vi "Facade.vi"(0 "Data In":T6, 2 "Display State In":T4, 3 "Container State":T5) -> (6 "Data Out":T6, 7 "Display State Out":T4, 8 "Action":T3)   [LabVIEW 2016, in "Queued Listbox.xctl"]
uses:
  Queued Listbox.xctl
  Data.ctl
  <vilib>/_xctls/Container State.ctl
  State.ctl
  <vilib>/_xctls/Action.ctl
  Menu object array.ctl
  Menu object.ctl
  <vilib>/_xctls/XControlSupport.lvlib
panel:
  out "Error Out":errorcluster
  in  "Menu object array":T1 {"Object name" items=["Select one..."]}
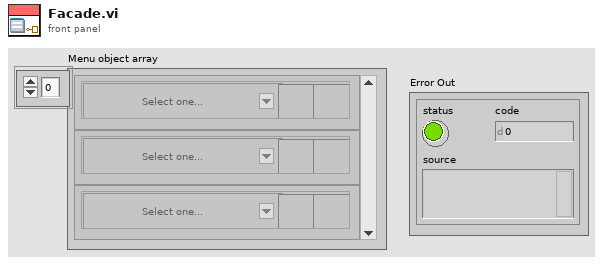
[diagram p1: front panel]
types:
  T1 = typedef "Menu object array.ctl" = T2[]
  T2 = typedef "Menu object.ctl" = cluster{"Object name":u16, "Open parameters":bool, "Remove Button":bool}
  T3 = typedef "XControlSupport.lvlib/Action.ctl" = cluster{"Data Changed?":bool, "State Changed?":bool, "Action Name":string}
  T4 = typedef "Queued Listbox.xctl/State.ctl" = cluster{"Strings":string[], "Selected items":i32[], "Message event":refnum<user-event>}
  T5 = typedef "XControlSupport.lvlib/Container State.ctl" = cluster{"Indicator?":bool, "Run Mode?":bool, " Refnum":refnum<vi>}
  T6 = typedef "Queued Listbox.xctl/Data.ctl" = string[]
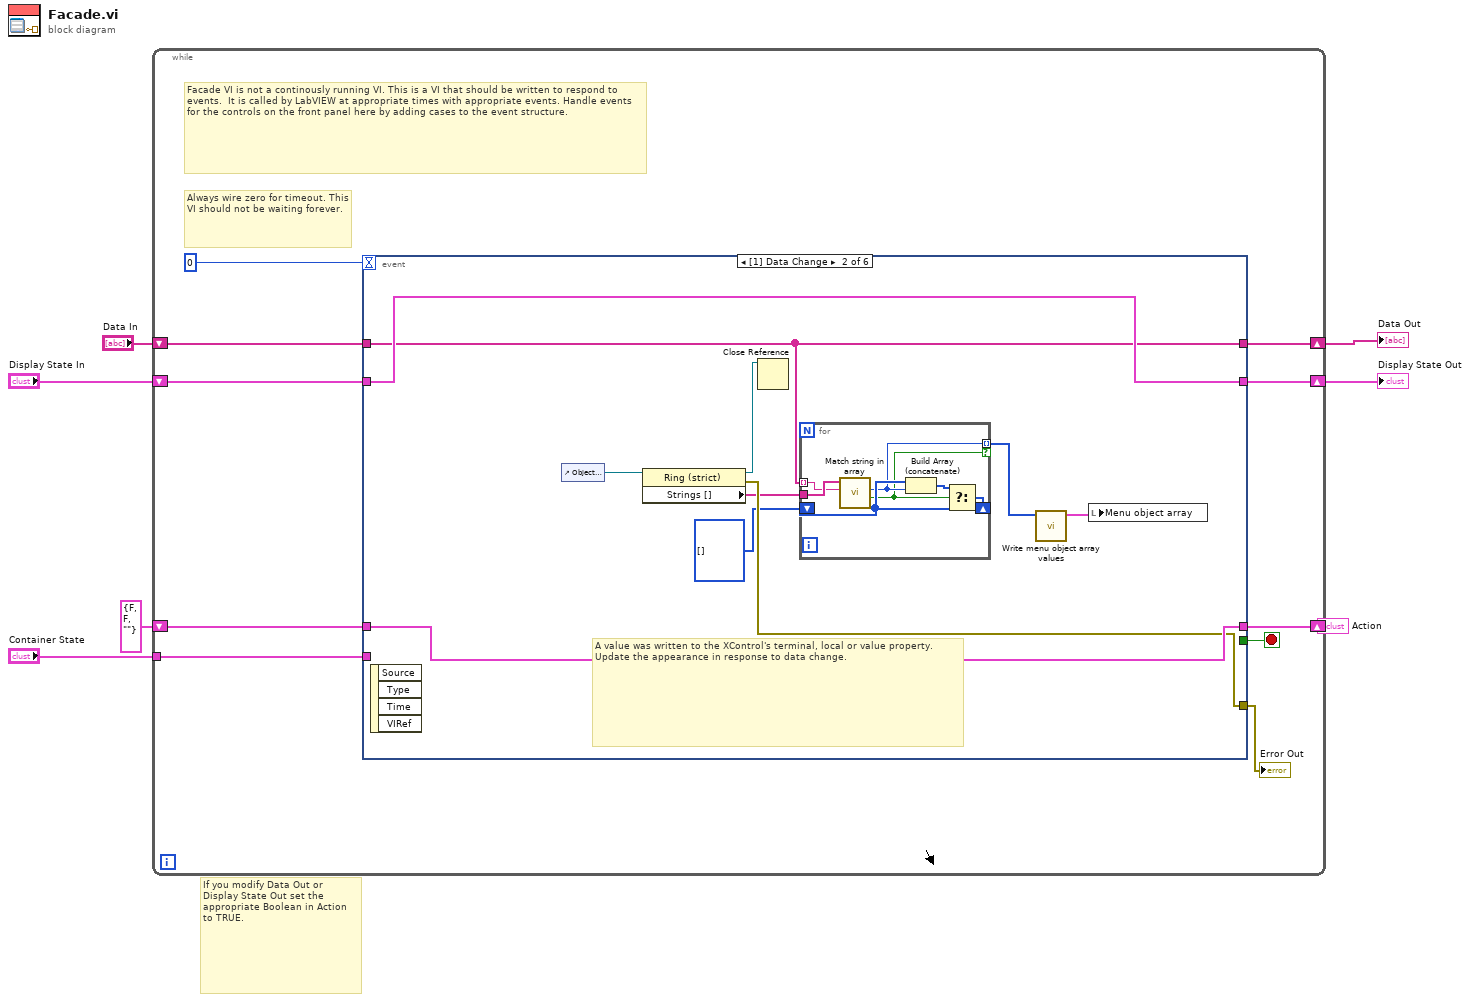
[diagram p0: block diagram]
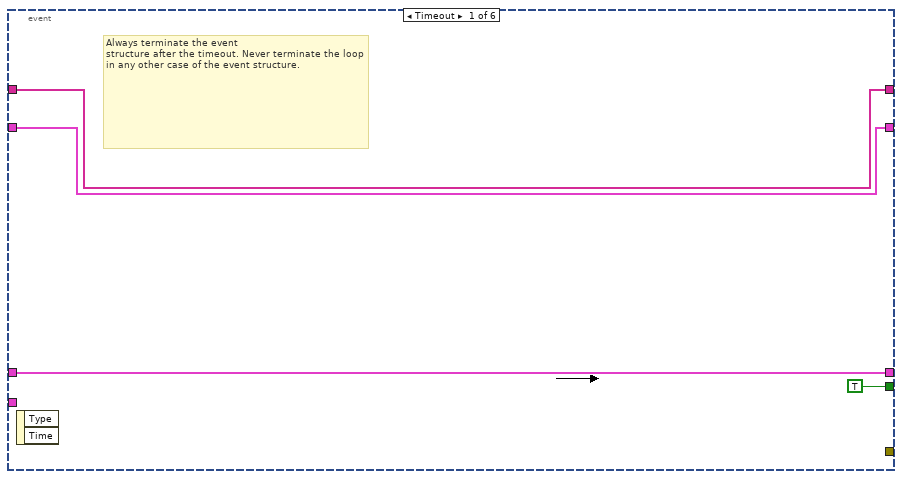
[diagram p2: hidden frame]
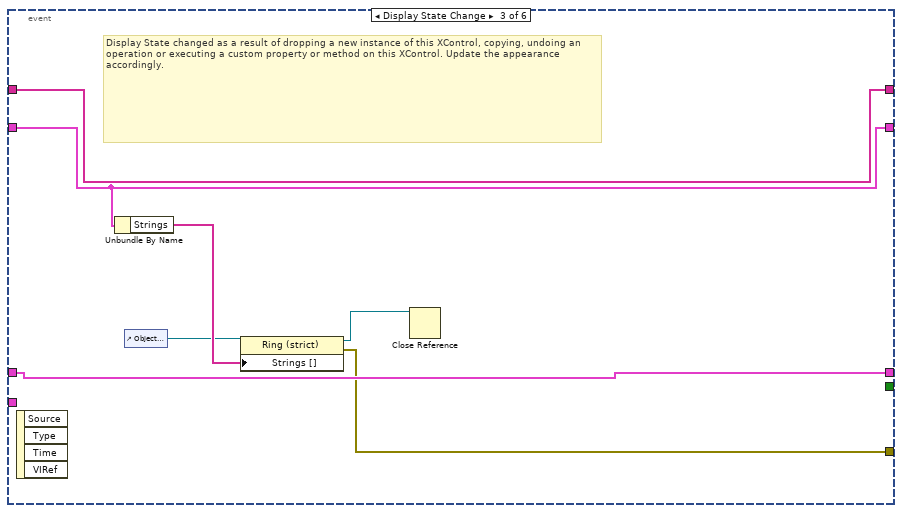
[diagram p3: hidden frame]
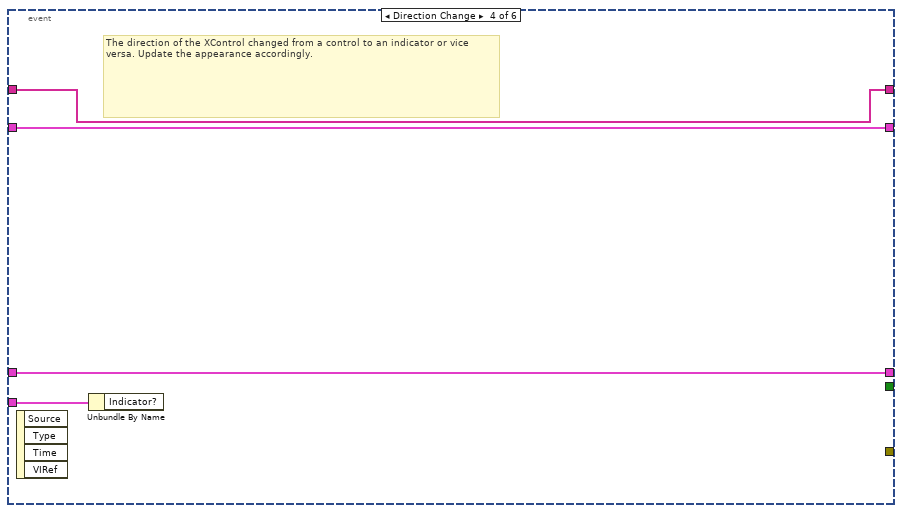
[diagram p4: hidden frame]
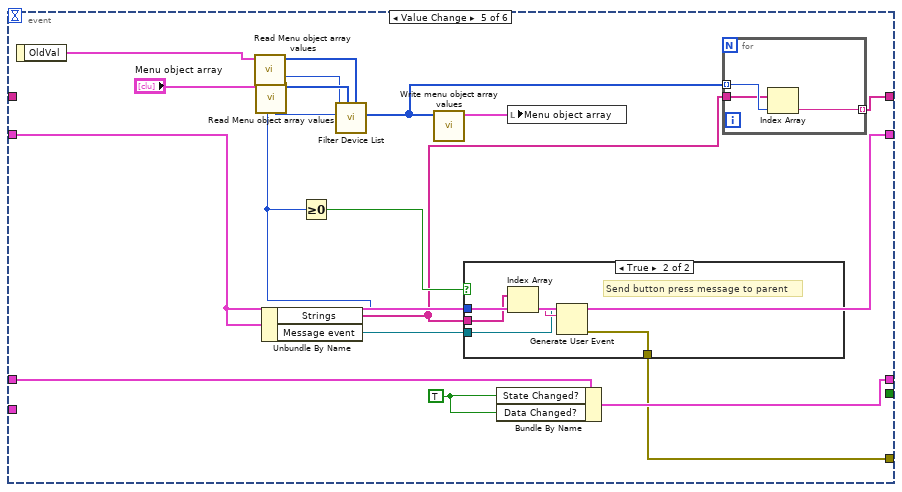
[diagram p5: hidden frame]
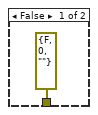
[diagram p6: hidden frame]
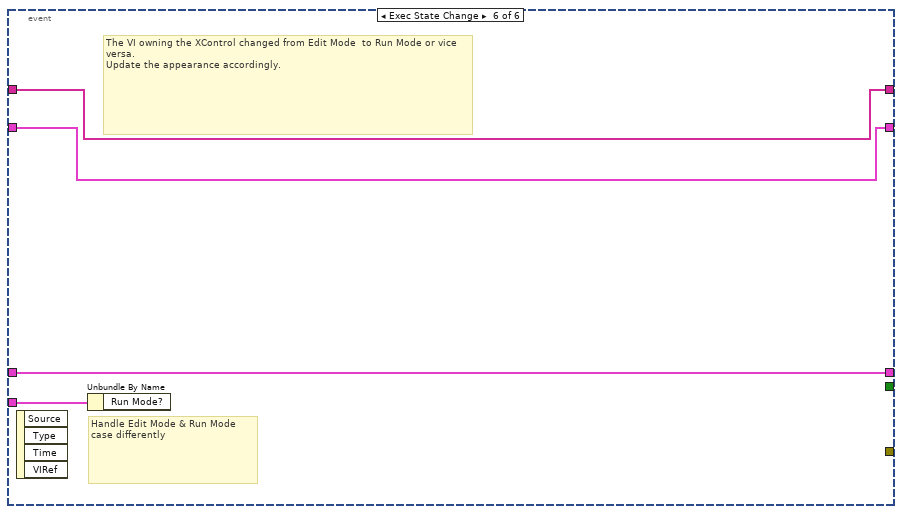
[diagram p7: hidden frame]
diagram:
  # "If you modify Data Out or\nDisplay State Out set the\nappropriate Boolean in Action\nto TRUE."
  n1 = while {
    shift-right: [w16] -> w4
    shift-left: "Display State In" -> [w17]
    tunnel: "Container State" -> [w13]
    shift-right: [w11] -> w7
    shift-left: "Data In" -> [w12]
    shift-right: [w9] -> w2
    shift-left: T3 {"Data Changed?"=FALSE, "State Changed?"=FALSE, "Action Name"=""} ("Action") -> [w10]
    stop <- w15 stop-if-true
    # "Facade VI is not a continously running VI. This is a VI that should be written to respond to events.  It is called by LabVIEW at appropriate times with appropriate events. Handle events for the controls on the front panel here by adding cases to the event structure."
    # "Always wire zero for timeout. This\nVI should not be waiting forever."
    n2 = event shown="[1] Data Change" {
      selector: _ -> [_ _ _ _ _ _]
      dyn-events: _ -> [_ _ _ _ _ _]
      timeout: 0 -> [_ _ _ _ _ _]
      tunnel: w17 -> [w19 w30 w40 w48 w63 w79]
      tunnel: [w19 w30 w40 w48 w63 w79] -> w16
      tunnel: [TRUE _ _ _ _ _] -> w15
      tunnel: w13 -> [_ _ _ w49 _ w80]
      tunnel: w12 -> [w18 w26 w45 w47 _ w78]
      tunnel: [w18 w26 w45 w47 w58 w78] -> w11
      tunnel: [w20 w31 w44 w46 w56 w77] -> w9
      tunnel: w10 -> [w20 w31 w44 w46 w67 w77]
      tunnel: [_ w29 w39 _ w54 _] -> w8
      event Timeout {
        # "Always terminate the event\nstructure after the timeout. Never terminate the loop in any other case of the event structure."
        n3 = event-data() -> ()  [unwired: 1 in, 2 out]
      }
      event Data Change {
        # "A value was written to the XControl's terminal, local or value property.\nUpdate the appearance in response to data change."
        n4 = event-data() -> ()  [unwired: 1 in, 4 out]
        n5 = control-ref of="Object name"() -> (w28:refnum<vi>)
        n6 = property class="Ring (strict)"(reference=w28) -> (reference out=w27:refnum<vi>, error out=w29:errorcluster, "Strings []"=w25:string[])  [unwired: 1 in]
        n7 = Close Reference(reference=w27) -> ()  [unwired: 1 in, 1 out]
        n8 = for {
          tunnel: w26 -> [w34] mode=indexing
          tunnel: w25 -> [w35]
          shift-right: [w36] -> _
          shift-left: i32[] [] -> [w37]
          tunnel: [w33] -> w22 mode=indexing if=w32
          n9 = call "Match string in array.vi"("String"=w34, "String Array"=w35) -> ("Found"=w32:bool, "Index"=w33:i32)  [unwired: 7 in, 1 out]
          n10 = Build Array (concatenate)(w37, w33) -> (w38:i32[])
          n11 = Select(t=w38, s=w32, f=w37) -> (s? t:f=w36:i32[])
        }
        n12 = call "Write menu object array values.vi"("Values"=w22) -> ("Menu object array"=w23:T1)  [unwired: 10 in]
        n13 = local write "Menu object array"(w23) -> ()
      }
      event Display State Change {
        # "Display State changed as a result of dropping a new instance of this XControl, copying, undoing an operation or executing a custom property or method on this XControl. Update the appearance accordingly."
        n14 = event-data() -> ()  [unwired: 1 in, 4 out]
        n15 = Unbundle By Name(w40) -> ("Strings"=w43:string[])
        n16 = control-ref of="Object name"() -> (w41:refnum<vi>)
        n17 = property class="Ring (strict)"(reference=w41, "Strings []"=w43) -> (reference out=w42:refnum<vi>, error out=w39:errorcluster)  [unwired: 1 in]
        n18 = Close Reference(reference=w42) -> ()  [unwired: 1 in, 1 out]
      }
      event Direction Change {
        # "The direction of the XControl changed from a control to an indicator or vice versa. Update the appearance accordingly."
        n19 = event-data() -> ()  [unwired: 1 in, 4 out]
        n20 = Unbundle By Name(w49) -> ()  [unwired: 1 out]
      }
      event Value Change {
        w55 = TRUE ("State Changed?")
        n21 = event-data() -> ("OldVal"=w65:T1)  [unwired: 1 in]
        n22 = call "Read Menu object array values.vi"("Menu object array"=w65) -> ("Values"=w64:u16[])  [unwired: 6 in, 4 out]
        n23 = call "Read Menu object array values.vi"("Menu object array"="Menu object array") -> ("Values"=w59:u16[], "Remove object pressed"=w51:i32, "Remove object"=w50:i32, "Open parameters for object"=w53:i32)  [unwired: 6 in, 1 out]
        n24 = Unbundle By Name(w63) -> ("Strings"=w57:string[], "Message event"=w62:refnum<user-event>)
        n25 = Greater Or Equal To 0?(x=w53) -> (x >= 0?=w60:bool)
        n26 = call "Filter Device List.vi"("Old List"=w64, "New List"=w59, "Remove object pressed"=w51, "Remove object"=w50) -> ("Filtered List"=w52:u16[])  [unwired: 7 in]
        n27 = call "Write menu object array values.vi"("Values"=w52) -> ("Menu object array"=w61:T1)  [unwired: 10 in]
        n28 = case shown="True" w60 {
          tunnel: w53 -> [_ w76]
          tunnel: w62 -> [_ w74]
          tunnel: w57 -> [_ w73]
          tunnel: [errorcluster {"status"=FALSE, "code"=0, "source"=""} ("error out") w72] -> w54
          frame False {
          }
          frame True {
            # "Send button press message to parent"
            n29 = Index Array(array=w73, index=w76) -> (element=w75:string)
            n30 = Generate User Event(user event=w74, event data cluster=w75) -> (error out=w72:errorcluster)  [unwired: 2 in, 1 out]
          }
        }
        n31 = Bundle By Name(cluster=w67, "State Changed?"=w55, "Data Changed?"=w55) -> (w56:T3)
        n32 = local write "Menu object array"(w61) -> ()
        n33 = for {
          tunnel: w52 -> [w70] mode=indexing
          tunnel: w57 -> [w69]
          tunnel: [w68] -> w58 mode=indexing
          n34 = Index Array(array=w69, index=w70) -> (element=w68:string)
        }
      }
      event Exec State Change {
        # "The VI owning the XControl changed from Edit Mode  to Run Mode or vice versa.\nUpdate the appearance accordingly."
        # "Handle Edit Mode & Run Mode\ncase differently"
        n35 = event-data() -> ()  [unwired: 1 in, 4 out]
        n36 = Unbundle By Name(w80) -> ()  [unwired: 1 out]
      }
    }
    "Error Out" <- w8
  }
  "Display State Out" <- w4
  "Data Out" <- w7
  "Action" <- w2
